vi "trame_ana.vi"(10 "OKdém?":bool, 11 "Chaîne":string) -> (3 "Instruction":string)   [LabVIEW 2020]
doc: "Analyse la trame pour voir dans quel cas on bacsule"
uses:
  <vilib>/regexp/Match Regular Expression.xnode
panel:
  out "error out":errorcluster
  in  "errin":errorcluster
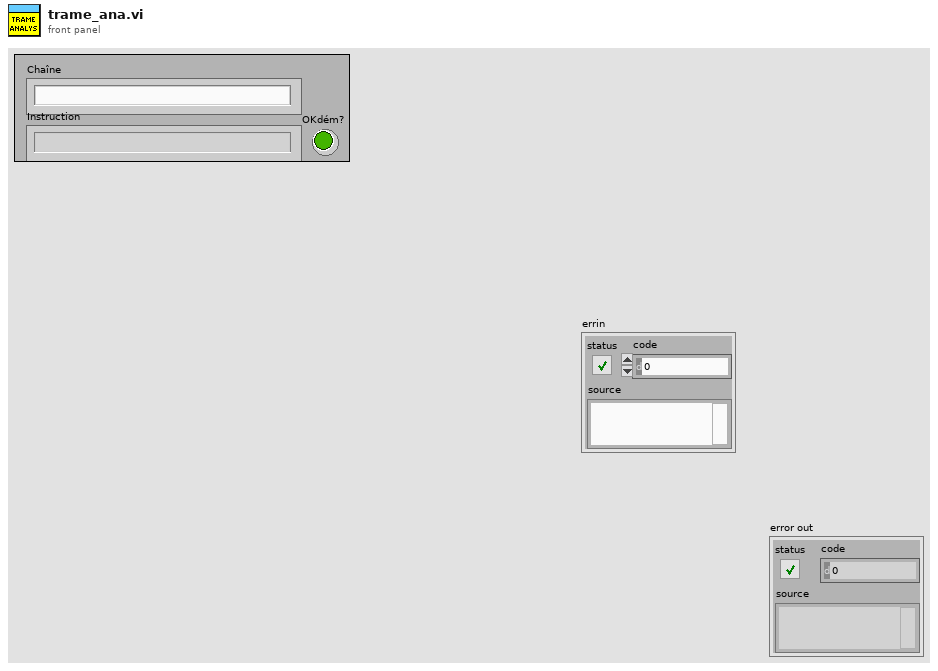
[diagram p1: front panel]
types:
  T1 = enum16{"open", "replace", "create", "open or create", "replace or create", "replace or create with confirmation"}
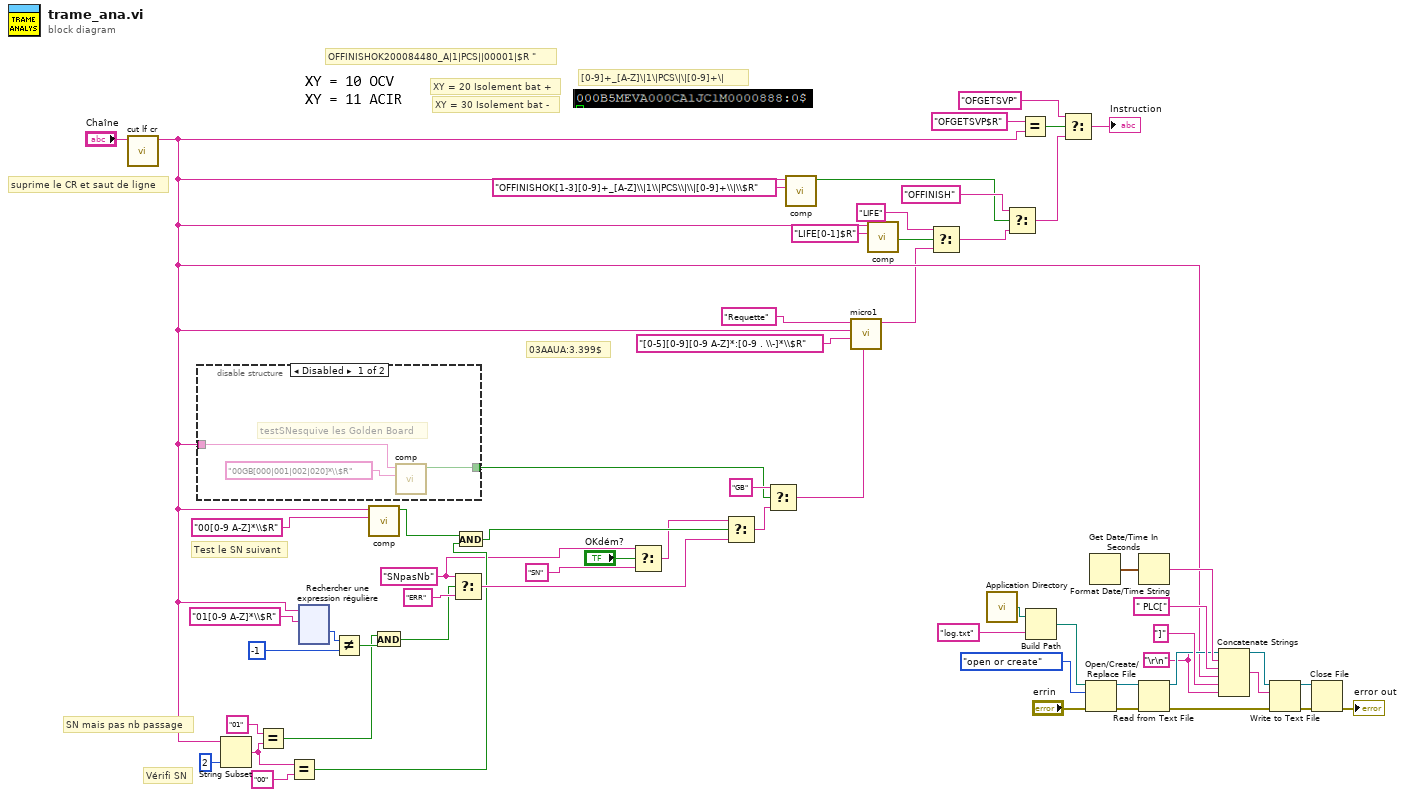
[diagram p0: block diagram]
diagram:
  w8 = "\r\n"
  w36 = "SNpasNb" ("cas vrai")
  # "[0-9]+_[A-Z]\\|1\\|PCS\\|\\|[0-9]+\\|"
  # "OFFINISHOK200084480_A|1|PCS||00001|$R \""
  # "Vérifi SN"
  # "SN mais pas nb passage"
  # "XY = 30 Isolement bat -"
  # "XY = 20 Isolement bat +"
  # "Test le SN suivant"
  # "suprime le CR et saut de ligne"
  # "03AAUA:3.399$"
  n1 = call "cut lf cr.vi"("strin"="Chaîne") -> ("strout"=w6:string)  [unwired: 10 in]
  n2 = disable-structure shown="Disabled" {
    disable-tunnel: [w62 _] -> w30
    disable-tunnel: w6 -> [w60 _]
    frame Disabled {
      # "testSNesquive les Golden Board"
      n3 = call "comp.vi"("expression régulière"="00GB[000|001|002|020]*\\$R", "strout"=w60) -> ("Boolean"=w62:bool)  [unwired: 9 in]
    }
    frame Enabled {
    }
  }
  n4 = String Subset ("Sous-ensemble d'une chaîne")(string=w6, length (rest)=2 ("longueur (reste)")) -> (substring=w43:string)  [unwired: 1 in]
  n5 = Equal? ("Égaux ?")(x="01", y=w43) -> (x = y?=w46:bool)
  n6 = Equal? ("Égaux ?")(x=w43, y="00") -> (x = y?=w41:bool)
  n7 = xnode "Rechercher une expression régulière"("chaîne en entrée"=w6, "expression régulière"="01[0-9 A-Z]*\\$R") -> ("offset après correspondance"=w50:i32)  [unwired: 4 in, 4 out]
  n8 = Not Equal? ("Différents ?")(x=w50, y=-1) -> (x != y?=w49:bool)
  n9 = call "comp.vi"("expression régulière"="00[0-9 A-Z]*\\$R", "strout"=w6) -> ("Boolean"=w29:bool)  [unwired: 9 in]
  n10 = And(x=w46, y=w49) -> (x .and. y?=w45:bool)
  n11 = Select ("Sélectionner")(t=w36, s=w45, f="ERR" ("cas faux")) -> (s? t:f=w53:string)
  n12 = And(x=w29, y=w41) -> (x .and. y?=w44:bool)
  n13 = Select ("Sélectionner")(t=w36, s="OKdém?", f="SN") -> (s? t:f=w37:string)
  n14 = Select ("Sélectionner")(t=w37, s=w44, f=w53) -> (s? t:f=w32:string)
  n15 = Select ("Sélectionner")(t="GB" ("cas vrai"), s=w30, f=w32) -> (s? t:f=w33:string)
  n16 = call "comp.vi"("expression régulière"="OFFINISHOK[1-3][0-9]+_[A-Z]\\|1\\|PCS\\|\\|[0-9]+\\|\\$R", "strout"=w6) -> ("Boolean"=w27:bool)  [unwired: 9 in]
  n17 = call "micro1.vi"("flux in en entrée"=w33, "expression régulière"="[0-5][0-9][0-9 A-Z]*:[0-9 . \\-]*\\$R", "data in"=w6, "cmd"="Requette") -> ("flux in en sortie"=w3:string)  [unwired: 7 in]
  n18 = call "comp.vi"("expression régulière"="LIFE[0-1]$R", "strout"=w6) -> ("Boolean"=w4:bool)  [unwired: 9 in]
  n19 = Select ("Sélectionner")(t="LIFE", s=w4, f=w3) -> (s? t:f=w2:string)
  n20 = call <vilib>:"Application Directory.vi"() -> ("Application Directory"=w24:path)
  n21 = Select ("Sélectionner")(t="OFFINISH", s=w27, f=w2) -> (s? t:f=w59:string)
  n22 = Equal? ("Égaux ?")(x="OFGETSVP$R", y=w6) -> (x = y?=w56:bool)
  n23 = Build Path ("Composer un chemin")(base path=w24, name or relative path="log.txt") -> (appended path=w23:path)
  n24 = Select(t="OFGETSVP", s=w56, f=w59) -> (s? t:f=→"Instruction":string)
  n25 = Open/Create/Replace File(file path (use dialog)=w23, error in="errin", operation (0:open)=T1."open or create") -> (refnum out=w11:refnum<file>, error out=w12:errorcluster)  [unwired: 3 in, 1 out]
  n26 = Get Date/Time In Seconds() -> (seconds since 1Jan1904=w17:timestamp)
  n27 = Format Date/Time String(seconds (now)=w17) -> (date/time string=w16:string)  [unwired: 2 in]
  n28 = Read from Text File(file (use dialog)=w11, error in=w12) -> (refnum out=w10:refnum<file>, error out=w13:errorcluster)  [unwired: 2 in, 2 out]
  n29 = Concatenate Strings(w8, w16, " PLC[" ("string"), w6, "]" ("string"), w8) -> (w9:string)
  n30 = Write to Text File(file (use dialog)=w10, text=w9, error in=w13) -> (refnum out=w18:refnum<file>, error out=w20:errorcluster)  [unwired: 1 in, 1 out]
  n31 = Close File(refnum=w18, error in=w20) -> (error out=→"error out":errorcluster)  [unwired: 1 out]
